vi "testDeltaPS.vi"() -> ()   [LabVIEW 2019]
panel:
  out "DeltaPS":string
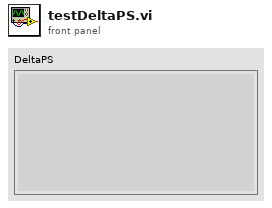
[diagram p1: front panel]
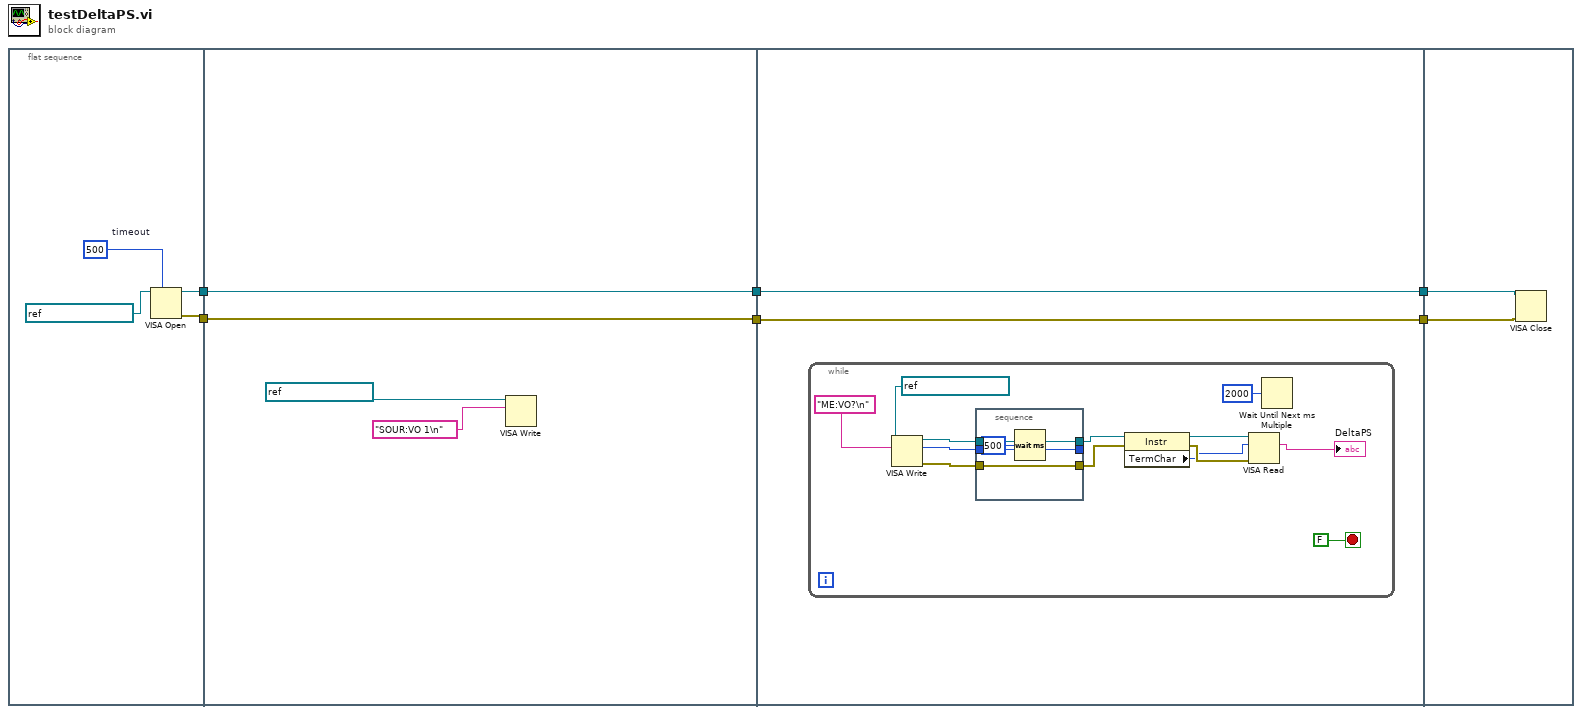
[diagram p0: block diagram]
diagram:
  n1 = flat-sequence {
    tunnel: [w8] -> w6
    tunnel: [w7] -> w5
    tunnel: w6 -> [w14]
    tunnel: w5 -> [w13]
    tunnel: [w14] -> w4
    tunnel: [w13] -> w2
    tunnel: w4 -> [w16]
    tunnel: [w16] -> w3
    tunnel: w2 -> [w15]
    tunnel: [w15] -> w1
    tunnel: w3 -> [w35]
    tunnel: w1 -> [w34]
    frame #0 {
      w9 = u32 500  # timeout
      n2 = VISA Open(timeout (0)=w9, VISA resource name=refnum<visa-resource-name> "GPIB0::8::INSTR") -> (VISA resource name=w8:refnum<visa-resource-name>, error out=w7:errorcluster)  [unwired: 3 in]
    }
    frame #1 {
      n3 = VISA Write(VISA resource name=refnum<visa-resource-name> "GPIB0::8::INSTR", write buffer="SOUR:VO 1\n") -> ()  [unwired: 1 in, 3 out]
    }
    frame #2 {
      n4 = while {
        stop <- FALSE stop-if-true
        n5 = VISA Write(VISA resource name=refnum<visa-resource-name> "GPIB0::8::INSTR", write buffer="ME:VO?\n") -> (VISA resource name out=w25:refnum<visa-resource-name>, return count=w23:u32, error out=w24:errorcluster)  [unwired: 1 in]
        n6 = stacked-sequence {
          tunnel: [w32] -> _
          tunnel: w25 -> [w32]
          tunnel: w24 -> [w30]
          tunnel: w23 -> [w31]
          tunnel: [w32] -> w22
          tunnel: [w31] -> _
          tunnel: [w30] -> w21
          frame #0 {
            n7 = Wait (ms)(milliseconds to wait=u32 500) -> ()  [unwired: 1 out]
          }
        }
        n8 = property class="Instr"(reference=w22, error in=w21) -> (reference out=w20:refnum<visa-resource-name>, error out=w19:errorcluster, "TermChar"=w18:u8)
        n9 = VISA Read(VISA resource name=w20, byte count=w18, error in (no error)=w19) -> (read buffer=→"DeltaPS":string)  [unwired: 3 out]
        n10 = Wait Until Next ms Multiple(millisecond multiple=u32 2000) -> ()  [unwired: 1 out]
      }
    }
    frame #3 {
      n11 = VISA Close(VISA resource name=w35, error in (no error)=w34) -> ()  [unwired: 1 out]
    }
  }
